vi "Data Manager.vi"(8 "error in (no error)":errorcluster, 9 "Mode":enum16{"Store Data", "Get Data", "Cleanup"}(ring)=enum."Get Data", 10 "Data In":T1 {"Transport Parameters"."Serial Communication"."Baud Rate" items=["75"=75, "110"=110, "134"=134, "150"=150, "300"=300, "600"=600, "1200"=1200, "1800"=1800, "2400"=2400, "4800"=4800, "7200"=7200, "9600"=9600, "14400"=14400, "19200"=19200, "28800"=28800, "38400"=38400, "56000"=56000, "57600"=57600, "115200"=115200, "128000"=128000, "230400"=230400]}, 11 "Refnum In":refnum<vi>) -> (0 "error out":errorcluster, 2 "Data Out":T1={"Transport Parameters"={"Serial Communication"={"Comport"="", "No Response Timeout Ms"=200, "Response Complete Timeout Ms"=1048, "Max Rx Length"=9600, "Baud Rate"=0}, "Selected Transport"=enum."Serial Communication Port", "Initializer File Path"=path "", "Cleaner File Path"=path "", "Transporter File Path"=path ""}, "Board Capabilities"={}} {"Transport Parameters"."Serial Communication"."Baud Rate" items=["75"=75, "110"=110, "134"=134, "150"=150, "300"=300, "600"=600, "1200"=1200, "1800"=1800, "2400"=2400, "4800"=4800, "7200"=7200, "9600"=9600, "14400"=14400, "19200"=19200, "28800"=28800, "38400"=38400, "56000"=56000, "57600"=57600, "115200"=115200, "128000"=128000, "230400"=230400]}, 3 "Refnum Out":refnum<vi>)   [LabVIEW 2020, in "FirmataClient.lvlib"]
doc: "All the data / state involved in the library is stored at a central point and hidden from the library. This VI must be used to interact with it (i.e. read, update or cleanup).\nThis state includes transport, connection information, board capability, ..."
uses:
  FirmataClient.lvlib
  Controls/Parameters.ctl
  Controls/TransportParameters.ctl
  Controls/SupportedTransports.ctl
  Controls/FirmataPinCapabilitiesAndAnalogMapping.ctl
  Controls/FirmataPinCapability.ctl
  Controls/FirmataPinModes.ctl
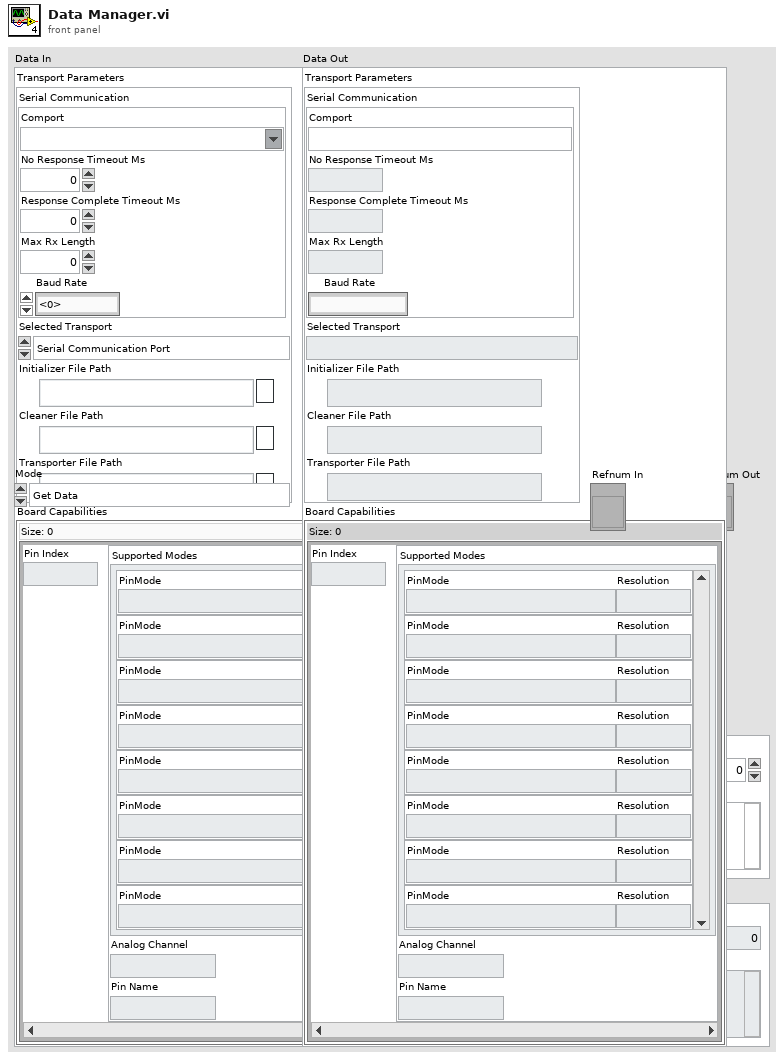
[diagram p1: front panel]
types:
  T1 = typedef "FirmataClient.lvlib/Parameters.ctl" = cluster{"Transport Parameters":T2, "Board Capabilities":map{i32, T4}}
  T2 = typedef "FirmataClient.lvlib/TransportParameters.ctl" = cluster{"Serial Communication":cluster{"Comport":refnum<visa-resource-name>, "No Response Timeout Ms":u32, "Response Complete Timeout Ms":u32, "Max Rx Length":u32, "Baud Rate":u32}, "Selected Transport":T3, "Initializer File Path":path, "Cleaner File Path":path, "Transporter File Path":path}
  T3 = typedef "FirmataClient.lvlib/SupportedTransports.ctl" = enum16{"Serial Communication Port"}
  T4 = typedef "FirmataClient.lvlib/FirmataPinCapabilitiesAndAnalogMapping.ctl" = cluster{"Supported Modes":T5[], "Analog Channel":u8, "Pin Name":string}
  T5 = typedef "FirmataClient.lvlib/FirmataPinCapability.ctl" = cluster{"PinMode":T6, "Resolution":u8}
  T6 = typedef "FirmataClient.lvlib/FirmataPinModes.ctl" = enum16{"DigitalInput", "DigitalOutput", "AnalogInput", "PWM", "Servo", "Shift", "I2C", "OneWire", "Stepper", "Encoder", "Serial", "InputPullup", "Extended.SPI", "Extended.Sonar", "Extended.Tone", "Extended.DHT"}
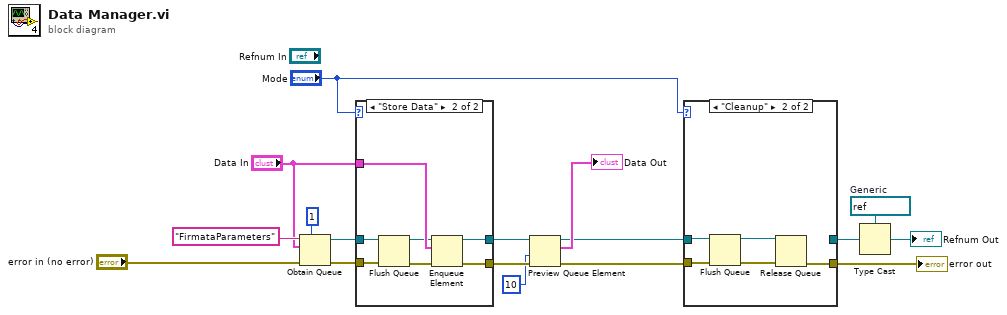
[diagram p0: block diagram]
diagram:
  w14 = refnum<vi> refnum  # Generic
  n1 = Obtain Queue(max queue size (-1, unlimited)=1, name (unnamed)="FirmataParameters", element data type="Data In", error in (no error)="error in (no error)") -> (queue out=w12:refnum<queue>, error out=w16:errorcluster)  [unwired: 1 in, 1 out]
  n2 = case shown="\"Store Data\"" "Mode" {
    tunnel: w16 -> [w18 w22]
    tunnel: "Data In" -> [_ w26]
    tunnel: w12 -> [w19 w23]
    tunnel: [w18 w25] -> w10
    tunnel: [w19 w24] -> w9
    frame Default {
    }
    frame "Store Data" {
      n3 = Flush Queue(queue=w23, error in (no error)=w22) -> (queue out=w21:refnum<queue>, error out=w20:errorcluster)  [unwired: 1 out]
      n4 = Enqueue Element(queue=w21, element=w26, error in (no error)=w20) -> (queue out=w24:refnum<queue>, error out=w25:errorcluster)  [unwired: 1 in, 1 out]
    }
  }
  n5 = Preview Queue Element(queue=w9, timeout in ms (-1)=10, error in (no error)=w10) -> (queue out=w7:refnum<queue>, element=→"Data Out":T1, error out=w6:errorcluster)  [unwired: 1 out]
  n6 = case shown="\"Cleanup\"" "Mode" {
    tunnel: w6 -> [w27 w32]
    tunnel: w7 -> [w28 w30]
    tunnel: [w27 w33] -> w5
    tunnel: [w28 _] -> w4
    frame Default {
    }
    frame "Cleanup" {
      n7 = Flush Queue(queue=w30, error in (no error)=w32) -> (queue out=w29:refnum<queue>, error out=w31:errorcluster)  [unwired: 1 out]
      n8 = Release Queue(queue=w29, error in (no error)=w31) -> (error out=w33:errorcluster)  [unwired: 1 in, 2 out]
    }
  }
  "error out" <- w5
  n9 = Type Cast(type=w14, x=w4) -> (*(type *) &x=→"Refnum Out":refnum<vi>)
